vi "DSF Configuration File to Cluster.vi"(8 "error in (no error)":errorcluster, 11 "dsf configuration file path":path) -> (0 "error out":errorcluster, 2 "framework configuration out":T1, 3 "dsf configuration file path dup":path)   [LabVIEW 2017, in "DSF Core.lvlib" / "Configuration Session.lvclass"]
uses:
  Configuration Session.lvclass
  Read Settings.vi
  Typedefs/DSF Engine Channel Configuration.ctl
  DSF Core.lvlib
  Typedefs/DSF Engine Transfer Configuration.ctl
  Typedefs/DSF Engine Transfer Group Configuration.ctl
  Typedefs/DSF Engine Plugin Configuration.ctl
  Typedefs/DSF Engine Framework Configuration.ctl
  Typedefs/DSF Settings Info.ctl
  Typedefs/DSF Timing Info.ctl
  Typedefs/DSF Byte Order.ctl
  Typedefs/DSF Data Type.ctl
  Typedefs/DSF Direction.ctl
  Typedefs/DSF Engine Plugin Thread Configuration.ctl
  Typedefs/DSF Timeout Behavior.ctl
  Read Plugin.vi
  Read All Plugin IDs.vi
  Read Transfer.vi
  Read Channel.vi
  Read Group.vi
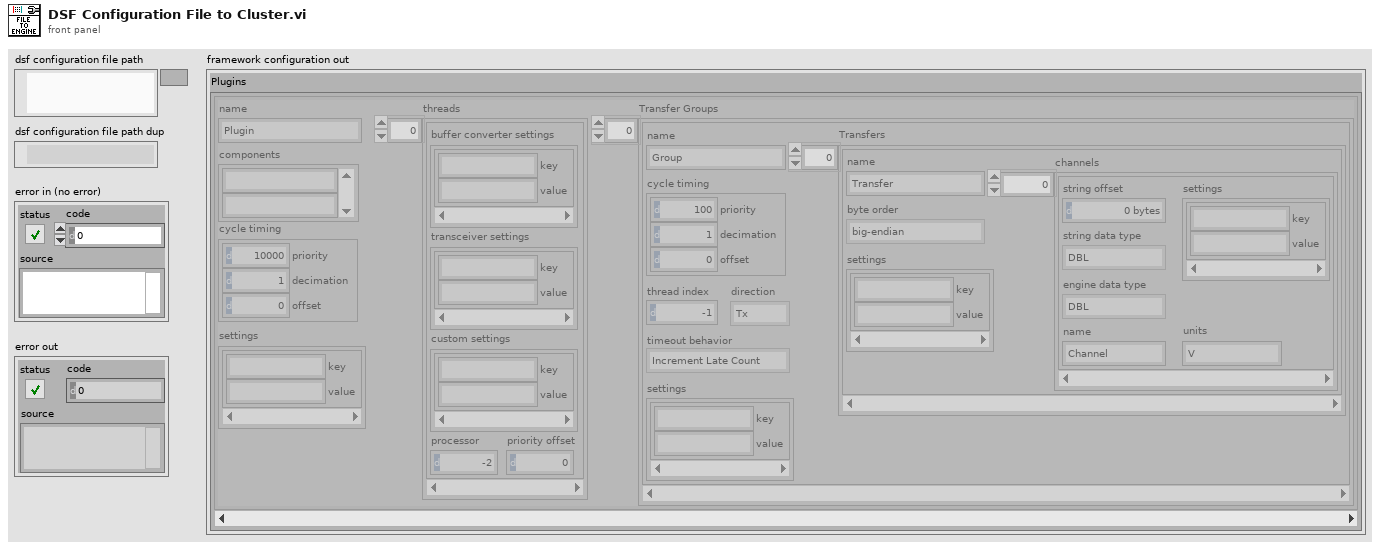
[diagram p1: front panel]
types:
  T1 = typedef "DSF Core.lvlib/DSF Engine Framework Configuration.ctl" = cluster{"Plugins":T2[]}
  T2 = typedef "DSF Core.lvlib/DSF Engine Plugin Configuration.ctl" = cluster{"name":string, "components":string[], "cycle timing":T3, "threads":T4[], "Transfer Groups":T6[], "settings":T5}
  T3 = typedef "DSF Core.lvlib/DSF Timing Info.ctl" = cluster{"priority":u64, "decimation":u64, "offset":u64}
  T4 = typedef "DSF Core.lvlib/DSF Engine Plugin Thread Configuration.ctl" = cluster{"buffer converter settings":T5, "transceiver settings":T5, "custom settings":T5, "processor":i32, "priority offset":i16}
  T5 = typedef "DSF Core.lvlib/DSF Settings Info.ctl" = cluster{"key":string, "value":string}[]
  T6 = typedef "DSF Core.lvlib/DSF Engine Transfer Group Configuration.ctl" = cluster{"name":string, "direction":T7, "cycle timing":T3, "thread index":i32, "settings":T5, "Transfers":T8[], "timeout behavior":T12}
  T7 = typedef "DSF Core.lvlib/DSF Direction.ctl" = enum8{"Tx", "Rx"}
  T8 = typedef "DSF Core.lvlib/DSF Engine Transfer Configuration.ctl" = cluster{"name":string, "byte order":T9, "settings":T5, "channels":T10[]}
  T9 = typedef "DSF Core.lvlib/DSF Byte Order.ctl" = enum8{"big-endian", "little-endian"}
  T10 = typedef "DSF Core.lvlib/DSF Engine Channel Configuration.ctl" = cluster{"string offset":u64, "string data type":T11, "engine data type":T11, "name":string, "settings":T5, "units":string}
  T11 = typedef "DSF Core.lvlib/DSF Data Type.ctl" = enum8{"Bool", "SGL", "DBL", "I8", "I16", "I32", "I64", "U8", "U16", "U32", "U64"}
  T12 = typedef "DSF Core.lvlib/DSF Timeout Behavior.ctl" = enum8{"Increment Late Count", "Throw Error"}
  T13 = typedef "DSF Core.lvlib/DSF Plugin Info.ctl" = cluster{"components":string[], "timing":T3, "group ids":string[], "settings id":string, "threads":T4[]}
  T14 = typedef "DSF Core.lvlib/DSF Group Info.ctl" = cluster{"direction":T7, "timing":T3, "transfer ids":string[], "settings id":string, "thread":i32, "timeout behavior":T12}
  T15 = typedef "DSF Core.lvlib/DSF Transfer Info.ctl" = cluster{"byte order":T9, "channel ids":string[], "settings id":string}
  T16 = typedef "DSF Core.lvlib/DSF Channel Info.ctl" = cluster{"string buffer offset":u64, "string data type":T11, "engine data type":T11, "settings id":string, "units":string}
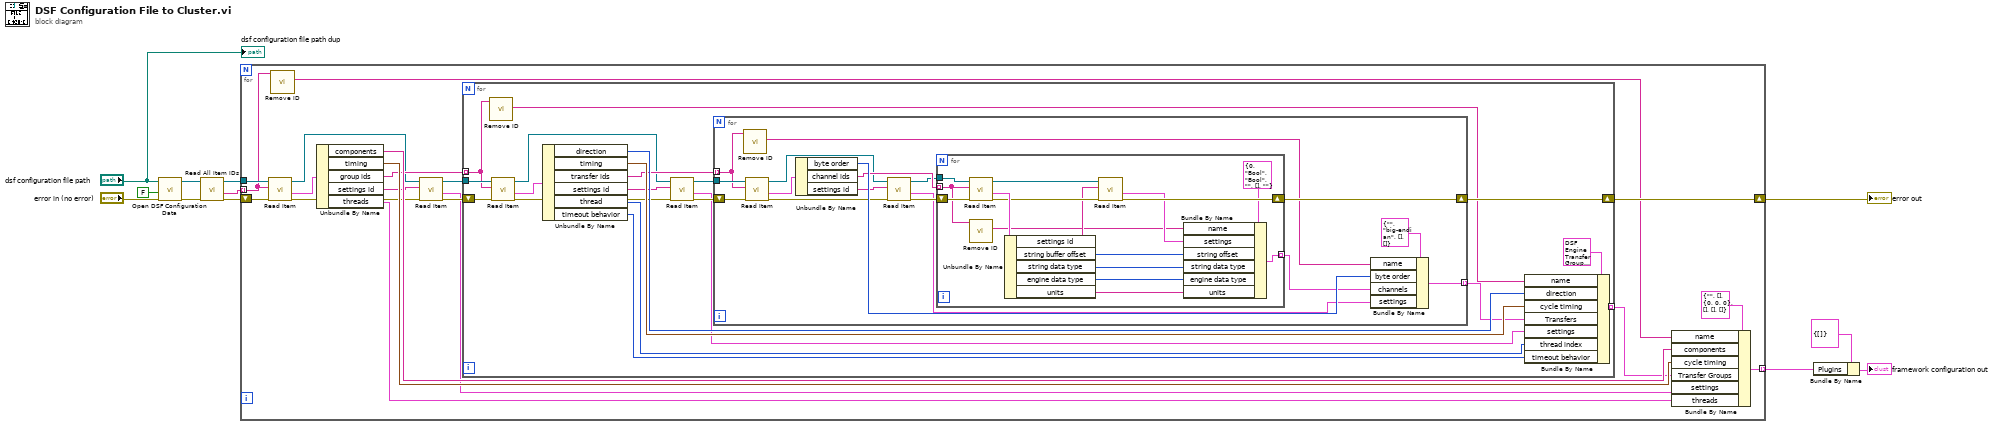
[diagram p0: block diagram]
diagram:
  n1 = call "Open DSF Configuration Data.vi"("error in (no error)"="error in (no error)", "replace if found? (F)"=FALSE ("create file if necessary (T)"), "dsf configuration file path"="dsf configuration file path") -> ("error out"=w5:errorcluster, "Configuration Session"=w6:refnum<class "Configuration Session.lvclass">)  [unwired: 4 in, 3 out]
  n2 = call-poly "Read All Item IDs.vi"("error in (no error)"=w5, "Configuration Session in"=w6) -> ("error out"=w1:errorcluster, "Plugin IDs"=w11:string[], "Configuration Session out"=w10:refnum<class "Configuration Session.lvclass">)  [unwired: 7 in]
  n3 = for {
    tunnel: w11 -> [w15] mode=indexing
    tunnel: w10 -> [w30]
    tunnel: [w26] -> w7 mode=indexing
    shift-right: [w18] -> w9
    shift-left: w1 -> [w13]
    n4 = call-poly "Read Item.vi"("error in (no error)"=w13, "Plugin ID"=w15, "Configuration Session in"=w30) -> ("error out"=w20:errorcluster, "value"=w29:T13, "Configuration Session out"=w23:refnum<class "Configuration Session.lvclass">)  [unwired: 5 in, 1 out]
    n5 = call "Remove ID.vi"("id string"=w15) -> ("name"=w14:string)  [unwired: 8 in, 2 out]
    n6 = Unbundle By Name(w29) -> ("components"=w28:string[], "timing"=w27:T3, "group ids"=w25:string[], "settings id"=w21:string, "threads"=w17:T4[])
    n7 = call-poly "Read Item.vi"("error in (no error)"=w20, "Settings ID"=w21, "Configuration Session in"=w23) -> ("error out"=w19:errorcluster, "value"=w16:T5, "Configuration Session out"=w22:refnum<class "Configuration Session.lvclass">)  [unwired: 5 in, 1 out]
    n8 = for {
      tunnel: w22 -> [w51]
      tunnel: w25 -> [w32] mode=indexing
      tunnel: [w46] -> w24 mode=indexing
      shift-right: [w36] -> w18
      shift-left: w19 -> [w43]
      n9 = call "Remove ID.vi"("id string"=w32) -> ("name"=w33:string)  [unwired: 8 in, 2 out]
      n10 = call-poly "Read Item.vi"("error in (no error)"=w43, "Group ID"=w32, "Configuration Session in"=w51) -> ("error out"=w39:errorcluster, "value"=w49:T14, "Configuration Session out"=w42:refnum<class "Configuration Session.lvclass">)  [unwired: 5 in, 1 out]
      n11 = Unbundle By Name(w49) -> ("direction"=w48:T7, "timing"=w47:T3, "transfer ids"=w45:string[], "settings id"=w40:string, "thread"=w35:i32, "timeout behavior"=w34:T12)
      n12 = call-poly "Read Item.vi"("error in (no error)"=w39, "Settings ID"=w40, "Configuration Session in"=w42) -> ("error out"=w38:errorcluster, "value"=w37:T5, "Configuration Session out"=w41:refnum<class "Configuration Session.lvclass">)  [unwired: 5 in, 1 out]
      n13 = for {
        tunnel: w45 -> [w53] mode=indexing
        tunnel: w41 -> [w68]
        tunnel: [w65] -> w44 mode=indexing
        shift-right: [w55] -> w36
        shift-left: w38 -> [w61]
        n14 = call "Remove ID.vi"("id string"=w53) -> ("name"=w52:string)  [unwired: 8 in, 2 out]
        n15 = call-poly "Read Item.vi"("error in (no error)"=w61, "Transfer ID"=w53, "Configuration Session in"=w68) -> ("error out"=w59:errorcluster, "value"=w67:T15, "Configuration Session out"=w62:refnum<class "Configuration Session.lvclass">)  [unwired: 5 in, 1 out]
        n16 = Unbundle By Name(w67) -> ("byte order"=w66:T9, "channel ids"=w63:string[], "settings id"=w58:string)
        n17 = call-poly "Read Item.vi"("error in (no error)"=w59, "Settings ID"=w58, "Configuration Session in"=w62) -> ("error out"=w57:errorcluster, "value"=w56:T5, "Configuration Session out"=w60:refnum<class "Configuration Session.lvclass">)  [unwired: 5 in, 1 out]
        n18 = for {
          tunnel: [w84] -> w64 mode=indexing
          tunnel: w63 -> [w71] mode=indexing
          tunnel: w60 -> [w83]
          shift-right: [w78] -> w55
          shift-left: w57 -> [w81]
          n19 = call-poly "Read Item.vi"("error in (no error)"=w81, "Channel ID"=w71, "Configuration Session in"=w83) -> ("error out"=w79:errorcluster, "value"=w82:T16, "Configuration Session out"=w80:refnum<class "Configuration Session.lvclass">)  [unwired: 5 in, 1 out]
          n20 = call "Remove ID.vi"("id string"=w71) -> ("name"=w69:string)  [unwired: 8 in, 2 out]
          n21 = Unbundle By Name(w82) -> ("settings id"=w76:string, "string buffer offset"=w72:u64, "string data type"=w73:T11, "engine data type"=w74:T11, "units"=w70:string)
          n22 = call-poly "Read Item.vi"("error in (no error)"=w79, "Settings ID"=w76, "Configuration Session in"=w80) -> ("error out"=w78:errorcluster, "value"=w75:T5)  [unwired: 5 in, 2 out]
          n23 = Bundle By Name(cluster=T10 {"string offset"=0, "string data type"=enum."Bool", "engine data type"=enum."Bool", "name"="", "settings"=[], "units"=""} ("channel configurations"), "name"=w69, "settings"=w75, "string offset"=w72, "string data type"=w73, "engine data type"=w74, "units"=w70) -> (w84:T10)
        }
        n24 = Bundle By Name(cluster=T8 {"name"="", "byte order"=enum."big-endian", "settings"=[], "channels"=[]} ("Transfer Configuration"), "name"=w52, "byte order"=w66, "channels"=w64, "settings"=w56) -> (w65:T8)
      }
      n25 = Bundle By Name(cluster=T6 {"name"="", "direction"=enum."Tx", "cycle timing"={"priority"=0, "decimation"=0, "offset"=0}, "thread index"=0, "settings"=[], "Transfers"=[], "timeout behavior"=enum."Increment Late Count"} ("Transfer Group Configuration"), "name"=w33, "direction"=w48, "cycle timing"=w47, "Transfers"=w44, "settings"=w37, "thread index"=w35, "timeout behavior"=w34) -> (w46:T6)
    }
    n26 = Bundle By Name(cluster=T2 {"name"="", "components"=[], "cycle timing"={"priority"=0, "decimation"=0, "offset"=0}, "threads"=[], "Transfer Groups"=[], "settings"=[]} ("Plugin Configuration"), "name"=w14, "components"=w28, "cycle timing"=w27, "Transfer Groups"=w24, "settings"=w16, "threads"=w17) -> (w26:T2)
  }
  "error out" <- w9
  n27 = Bundle By Name(cluster=T1 {"Plugins"=[]} ("Framework Config (JSON)"), "Plugins"=w7) -> (→"framework configuration out":T1)
  "dsf configuration file path dup" <- "dsf configuration file path"
